vi "Queue_Create.vi"(8 "error in (no error)":errorcluster) -> (0 "error out":errorcluster, 3 "Queue out":refnum<queue>)   [LabVIEW 2018, in "HttpClient_NET.lvlib" / "HttpClient_NET.lvclass"]
doc: "<b> </b> <b> </b>\nHttpClient_NET\nJustin Young - Viviota\nCopyright (c) 2021\nLicense: BSD"
uses:
  HttpClient_NET.lvclass
  HttpResponseMessage/Types/ResponseMessage_Cluster.ctl
  HttpResponseMessage/HttpResponseMessage.lvclass
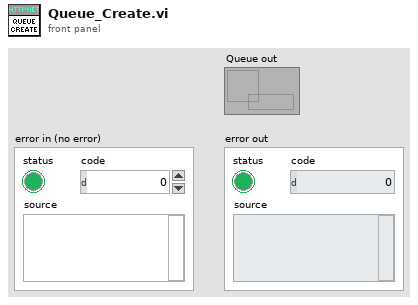
[diagram p1: front panel]
types:
  T1 = typedef "HttpClient_NET.lvlib/HttpResponseMessage.lvclass/ResponseMessage_Cluster.ctl" = cluster{"HttpResponseMessage":refnum<class "HttpResponseMessage.lvclass">, "TaskSuccess":bool}
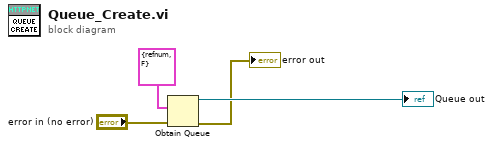
[diagram p0: block diagram]
diagram:
  n1 = Obtain Queue(element data type=T1 {"HttpResponseMessage"=refnum, "TaskSuccess"=FALSE} ("cluster"), error in (no error)="error in (no error)") -> (queue out=→"Queue out":refnum<queue>, error out=→"error out":errorcluster)  [unwired: 3 in, 1 out]
